vi "save.vi"() -> ()   [LabVIEW 2025]
panel:
  in  "Dial 3":dbl(knob) scale=0.0..10.0
  in  "Dial 2":dbl(knob) scale=0.0..10.0
  in  "Dial":dbl(knob) scale=0.0..10.0
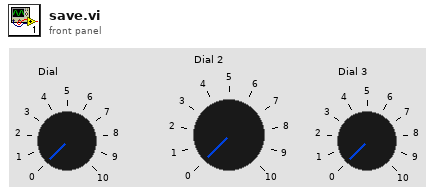
[diagram p1: front panel]
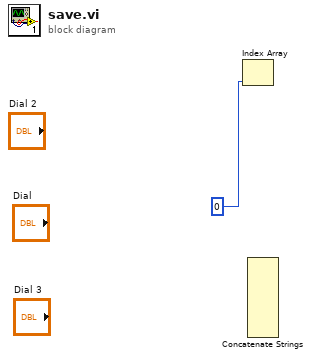
[diagram p0: block diagram]
diagram:
  n1 = Index Array(index=0) -> ()  [unwired: 1 in, 1 out]
  n2 = Concatenate Strings() -> ()  [unwired: 10 in, 1 out]
